vi "Get Resource Purpose.vi"(4 "Resource in":refnum<class "Resource.lvclass">) -> (7 "Resource Purpose":string)   [LabVIEW 2024, in "CTI.lvlib" / "Resource.lvclass"]
uses:
  Resource.lvclass
  Resource.lvclass/Resource.ctl
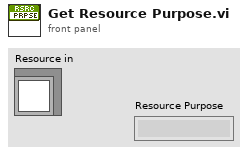
[diagram p1: front panel]
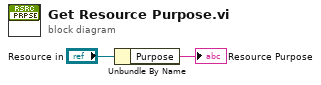
[diagram p0: block diagram]
diagram:
  n1 = Unbundle By Name("Resource in") -> ("Purpose"=→"Resource Purpose":string)
